vi "Generate Sequence.vi"(8 "error in (no error)":errorcluster, 11 "Toggle 6 in":refnum<class "Toggle 6.lvclass">) -> (0 "error out":errorcluster, 3 "Toggle 6 out":refnum<class "Toggle 6.lvclass">)   [LabVIEW 2020, in "Toggle 6.lvclass"]
doc: "Generates the test sequence and puts this into the class data"
uses:
  Toggle 6.lvclass
  C:/Sandbox/RF Bench/Source Code/WiSpry Test Framework/Devices/Device.lvclass
  Controls/Test Sequence.ctl
  Controls/Register to Write.ctl
  Controls/EFuse modes enum.ctl
  PIC-device/PIC-Device.lvclass
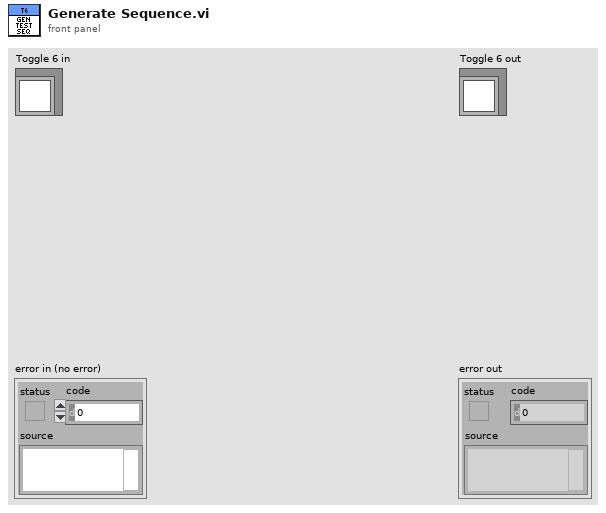
[diagram p1: front panel]
types:
  T1 = typedef "Toggle 6.lvclass/Test Sequence.ctl" = cluster{"Charge Pump Settings":T2[], "Charge Pump Values":dbl[], "Efuse Register Array":T2[], "Efuse Array":T3[], "Cap Register Array":T2[], "Cap Value Array":cluster{"Register Number":u32, "Value":dbl}[]}
  T2 = typedef "PIC-Device.lvclass/Register to Write.ctl" = cluster{"Register":u32, "Value":u32, "Dev Address":u32, "Physical Adress":u32}
  T3 = typedef "Toggle 6.lvclass/EFuse modes enum.ctl" = enum16{"On", "Off", "Both On and Off"}
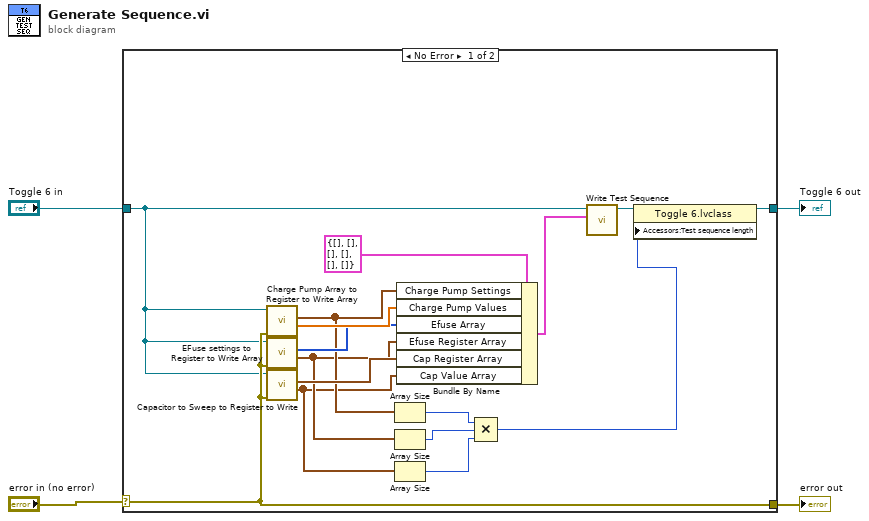
[diagram p0: block diagram]
diagram:
  n1 = case shown="No Error" "error in (no error)" {
    selector: "error in (no error)" -> [w20 w22]
    tunnel: [w20 w22] -> w3
    tunnel: [w5 w21] -> w1
    tunnel: "Toggle 6 in" -> [w15 w21]
    frame No Error {
      n2 = call "Charge Pump Array to Register to Write Array.vi"("error in (no error)"=w20, "Toggle 6 in"=w15) -> ("Charge Pump Values"=w19:dbl[], "Charge Pump Settings"=w13:T2[])  [unwired: 6 in, 2 out]
      n3 = call "EFuse settings to Register to Write Array.vi"("error in (no error)"=w20, "Toggle 6 in"=w15) -> ("Efuse Register Array"=w12:T2[], "Efuse Array"=w18:T3[])  [unwired: 6 in, 2 out]
      n4 = call "Capacitor to Sweep to Register to Write.vi"("error in (no error)"=w20, "Toggle 6 in"=w15) -> ("Cap Value Array"=w11:cluster{"Register Number":u32, "Value":dbl}[], "Cap Register Array"=w17:T2[])  [unwired: 6 in, 2 out]
      n5 = Array Size(array=w13) -> (size(s)=w10:i32)
      n6 = Array Size(array=w12) -> (size(s)=w9:i32)
      n7 = Array Size(array=w11) -> (size(s)=w8:i32)
      n8 = Bundle By Name(cluster=T1 {"Charge Pump Settings"=[], "Charge Pump Values"=[], "Efuse Register Array"=[], "Efuse Array"=[], "Cap Register Array"=[], "Cap Value Array"=[]}, "Charge Pump Settings"=w13, "Charge Pump Values"=w19, "Efuse Array"=w18, "Efuse Register Array"=w12, "Cap Register Array"=w17, "Cap Value Array"=w11) -> (w14:T1)
      n9 = Compound Arithmetic op=MULTIPLY(w10, w9, w8) -> (w6:i32)
      n10 = call-dynamic "Write Test Sequence.vi"("Test Sequence"=w14, "Toggle 6 in"=w15) -> ("Toggle 6 out"=w7:refnum<class "Toggle 6.lvclass">)  [unwired: 9 in]
      n11 = property class="Toggle 6.lvclass"(reference=w7, "Accessors:Test sequence length"=w6) -> (reference out=w5:refnum<class "Toggle 6.lvclass">)  [unwired: 1 in, 1 out]
    }
    frame Error {
    }
  }
  "error out" <- w3
  "Toggle 6 out" <- w1
